vi "Chemiluminescence_VI_BM.vi"(8 "BitNum":u32, 11 "BoardNum":u32=1) -> ()   [LabVIEW 2021]
uses:
  <vilib>/ULx/Create Channel.llb/ULx Create Channel (AI-Voltage-Basic).vi
  <vilib>/ULx/Read.llb/ULx Read (Analog DBL 1Chan 1Samp).vi
  <vilib>/express/express shared/transition.llb/Dynamic To Waveform Array.vi
  <vilib>/express/express signal manip/GetorSetDDTAttributes/Set DDT Attributes/SetT0.vi
  <vilib>/express/express shared/transition.llb/Waveform Array To Dynamic.vi
  <vilib>/express/express signal manip/GetorSetDDTAttributes/Set DDT Attributes/Set DDT Properties.xnode
  <vilib>/ptbypt/NI_PtbyPt.lvlib
  <vilib>/Analysis/NI_AALBase.lvlib
panel:
  in  "Integrate Peaks":bool
  in  "Drop pt.s?":i32=1
  in  "Width":i32=6
  in  "Window (s)":dbl=5.0
  in  "Plot Type":T1(ring)=enum."Raw Data"
  in  "stop":bool
  out "Stop indicator":bool
  out "error out":errorcluster
  in  "Tab Control":enum32{"Metadata", "Detector Params", "GPS"}(tab)
  out "Time Remaining":string="11:05:15"
  out "Iteration":i32=53112
  out "JD_Second":dbl=57.335 format="%_2g"
  out "JD_Hour":dbl=13.0 format="%_2g"
  out "JD_Minute":dbl=11.0 format="%_2g"
  out "Julian Day":dbl=47.54996527777778 format="%_14g"
  out "Latitude":dbl=5158.901913
  out "Longitude":dbl=11500.024835
  out "Day":dbl=47.0 format="%#_12g"
  out "Elapsed Time (s)":dbl=17685.58402299881
  in  "Format Date":string="%d-%d-%d"
  out "Date Output":string="2024-02-16"
  in  "max V":dbl=5.0
  in  "min V":dbl=-5.0
  in  "DAQ Type":u16(ring) items=["NI DAQ", "MC DAQ"]
  in  "Sampling Frequency":dbl=3.0
  in  "device name":tag="Dev1"
  in  "Runtime Limit (mins)":dbl=960.0 format="%#_13g"
  in  "GPS\nConnected?":bool=TRUE
  in  "GPS\n 2":refnum<visa-resource-name>="COM1"
  in  "GPS Baud":dbl=4800.0
  out "GPS_Latitude":dbl=5158.901913 format="%_4g"
  out "GPS_Longitude":dbl=11500.024835 format="%_4g"
  out "GPS_jd":dbl=47.54995370370371 format="%_5g"
  out "GPS_Day":dbl=47.0
  out "GPS_Hour":dbl=13.0
  out "GPS_Minute":dbl=11.0
  out "GPS_Second":dbl=56.0
  in  "Local save location:":string="C:\\Users\\LabPC1\\OneDrive\\Desktop\\CL_Data\\MISO\\CL_test"
  in  "Cruise ID":string="MISO"
  in  "Add a comment to file (MID)":string=" "
  in  "Backup save location:":string="C:\\Users\\LabPC1\\OneDrive\\Desktop\\CL_Backup_Data\\MISO\\CL_test"
  out "Windowed SD (V)":dbl=0.038392270385846874 format="%0.2f"
  out "Windowed Mean (V)":dbl=0.04536187144435753 format="%0.2f"
  out "PMT (V)":dbl=0.0252248007909035 format="%_6g"
  out "PMT V out":cluster{"Y":dbl[], "Y":dbl[]}[](graph)
  out "Hour":dbl=13.0
  out "Minute":dbl=11.0
  out "Second":dbl=11.0
  # "DMS/O/P Chemiluminescence Program"
  # "Hz"
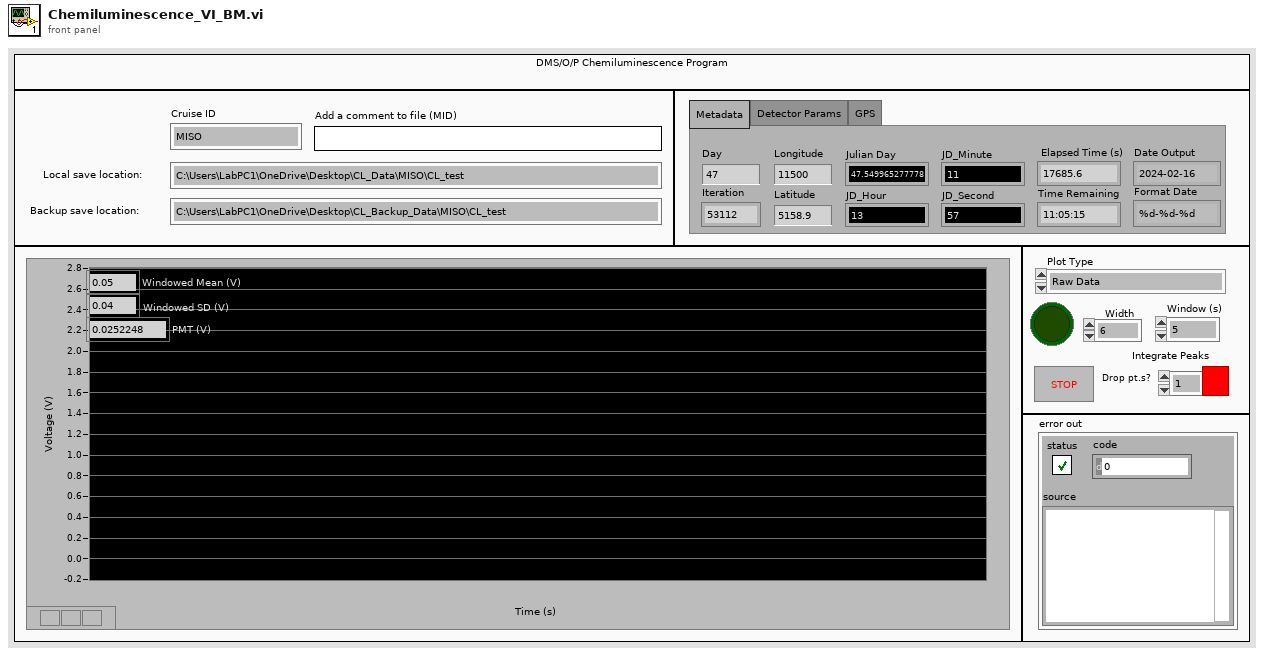
[diagram p1: front panel]
types:
  T1 = enum16{"Raw + Running Mean", "Running Mean", "Raw Data"}
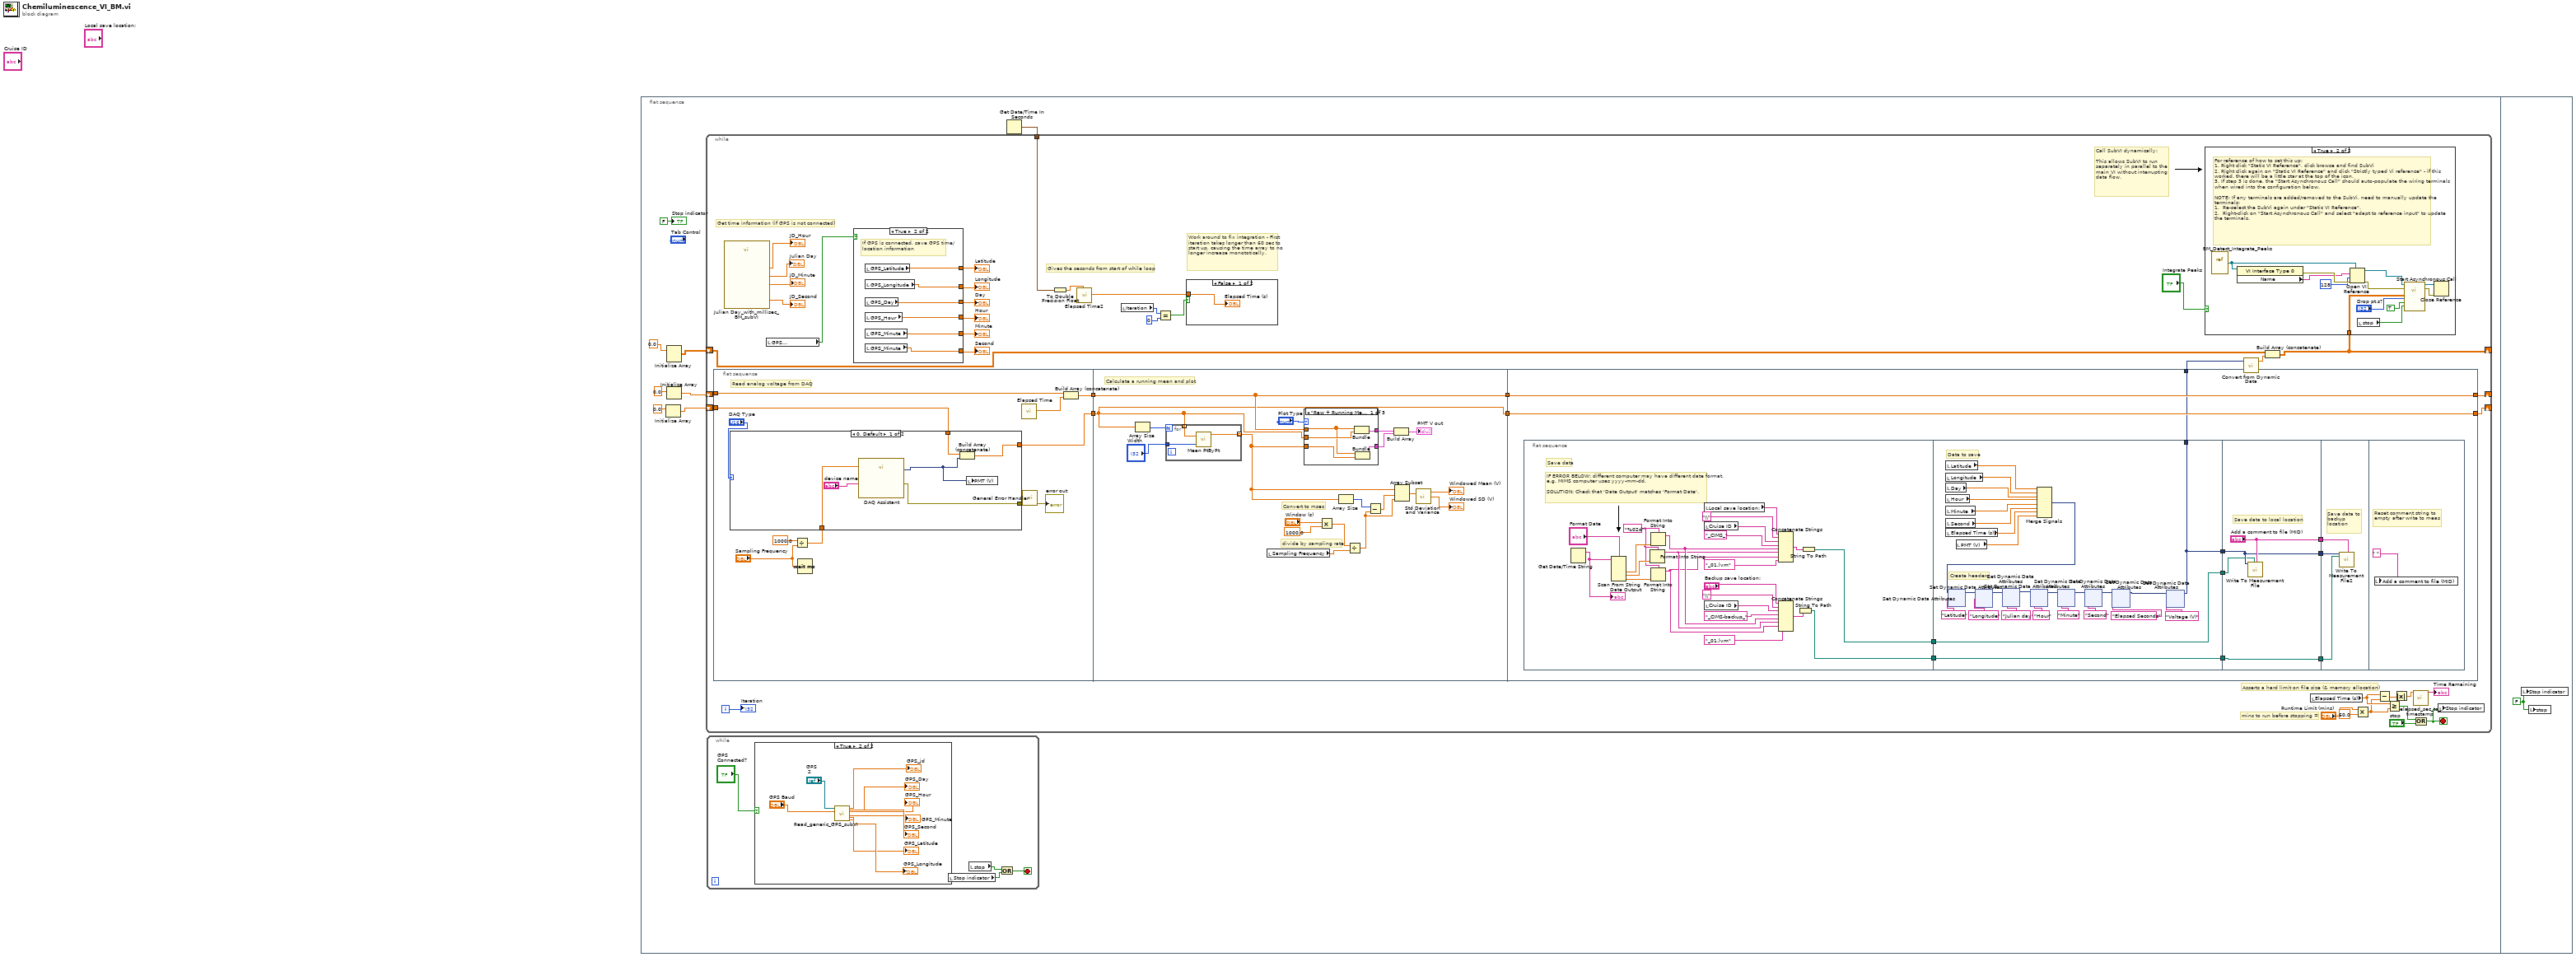
[diagram p0: block diagram]
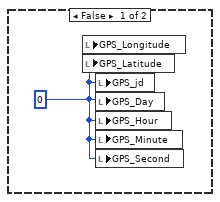
[diagram p2: hidden frame]
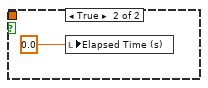
[diagram p4: hidden frame]
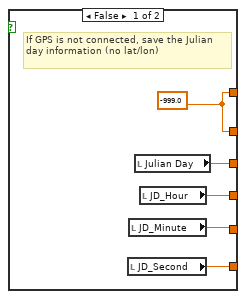
[diagram p5: hidden frame]
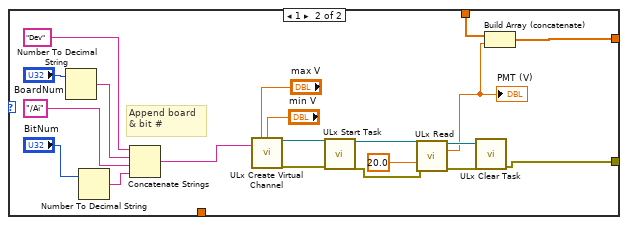
[diagram p6: hidden frame]
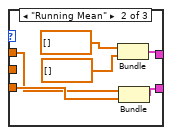
[diagram p7: hidden frame]
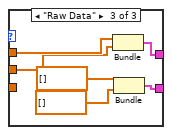
[diagram p8: hidden frame]
diagram:
  n1 = flat-sequence {
    frame #0 {
      n2 = Initialize Array(0.0 ("element")) -> (w5:dbl[])  [unwired: 1 in]
      n3 = Initialize Array(0.0 ("element")) -> (w1:dbl[][])  [unwired: 2 in]
      n4 = Initialize Array(0.0 ("element")) -> (w7:dbl[])  [unwired: 1 in]
      n5 = while {
        stop <- w10 stop-if-true
        n6 = case shown="True" "GPS\nConnected?" {
          frame False {
            w13 = 0
            n7 = local write "GPS_Longitude"(w13) -> ()
            n8 = local write "GPS_Latitude"(w13) -> ()
            n9 = local write "GPS_jd"(w13) -> ()
            n10 = local write "GPS_Day"(w13) -> ()
            n11 = local write "GPS_Hour"(w13) -> ()
            n12 = local write "GPS_Minute"(w13) -> ()
            n13 = local write "GPS_Second"(w13) -> ()
          }
          frame True {
            n14 = call "Read_generic_GPS_subVI.vi"("Baud Rate"="GPS Baud", "VISA resource name"="GPS\n 2") -> ("Longitude W"=→"GPS_Longitude":dbl, "GPS\nSeconds"=→"GPS_Second":dbl, "GPS\nHour"=→"GPS_Hour":dbl, "GPS JD"=→"GPS_jd":dbl, "Latitude N"=→"GPS_Latitude":dbl, "GPS\nDay"=→"GPS_Day":dbl, "GPS\nMinute"=→"GPS_Minute":dbl)  [unwired: 3 in]
          }
        }
        n15 = local read "Stop indicator"() -> (w9:bool)
        n16 = local read "stop"() -> (w11:bool)
        n17 = Or(x=w11, y=w9) -> (x .or. y?=w10:bool)
      }
      n18 = Get Date/Time In Seconds() -> (seconds since 1Jan1904=w4:timestamp)
      n19 = while {
        shift-right: [w28] -> _
        shift-left: w5 -> [w63]
        shift-right: [w61] -> _
        shift-left: w7 -> [w62]
        tunnel: w4 -> [w40]
        shift-right: [w23] -> _
        shift-left: w1 -> [w24]
        i -> [w32]
        stop <- w34 stop-if-true
        # "Call SubVI dynamically:\n\nThis allows SubVI to run separately in parallel to the main VI without interrupting data flow."
        # "mins to run before stopping ="
        # "Asserts a hard limit on file size (& memory allocation)"
        # "Work around to fix integration - First iteration takes longer than 60 sec to start up, causing the time array to no longer increase monototically."
        # "Gives the seconds from start of while loop"
        # "Get time information (if GPS is not connected)"
        n20 = flat-sequence {
          tunnel: w63 -> [w93]
          tunnel: w62 -> [w96]
          tunnel: [w92] -> w60
          tunnel: [w95] -> w58
          tunnel: w60 -> [w129]
          tunnel: [w129] -> w59
          tunnel: w58 -> [w143]
          tunnel: [w143] -> w57
          tunnel: [w175] -> w28
          tunnel: w59 -> [w175]
          tunnel: w57 -> [w174]
          tunnel: [w174] -> w61
          tunnel: [w165] -> w25
          frame #0 {
            # "Read analog voltage from DAQ"
            n21 = Divide(x=1000.0, y="Sampling Frequency") -> (x/y=w89:dbl)
            n22 = case shown="0, Default" "DAQ Type" {
              tunnel: [w104 w109] -> w99
              tunnel: w93 -> [w103 w108]
              tunnel: [w102 w107] -> w92
              tunnel: w89 -> [w100 _]
              frame 0, Default {
                n23 = call "DAQ Assistant"("number of samples"=w100, "device name"="device name") -> ("data"=w101:dynamicdata, "error out"=w104:errorcluster)  [unwired: 14 in, 2 out]
                n24 = Build Array (concatenate)(w103, w101) -> (w102:dbl[])
                n25 = local write "PMT (V)"(w101) -> ()
              }
              frame 1 {
                # "Append board\n& bit #"
                n26 = Number To Decimal String(number="BoardNum") -> (decimal integer string=w120:string)  [unwired: 1 in]
                n27 = Number To Decimal String(number="BitNum") -> (decimal integer string=w121:string)  [unwired: 1 in]
                n28 = Concatenate Strings("Dev", w120, "/Ai", w121) -> (w118:string)
                n29 = call-poly <vilib>:"ULx Create Virtual Channel.vi"("maximum value"="max V", "minimum value"="min V", "physical channels"=w118) -> ("task out"=w113:refnum<k24>, "error out"=w110:errorcluster)  [unwired: 11 in]
                n30 = call <vilib>:"ULx Start Task.vi"("task in"=w113, "error in"=w110) -> ("task out"=w112:refnum<k24>, "error out"=w111:errorcluster)  [unwired: 12 in]
                n31 = call-poly <vilib>:"ULx Read.vi"("task in"=w112, "timeout"=20.0, "error in"=w111) -> ("task out"=w125:refnum<k24>, "data"=w106:dbl, "error out"=w124:errorcluster)  [unwired: 10 in]
                "PMT (V)" <- w106
                n32 = call <vilib>:"ULx Clear Task.vi"("task in"=w125, "error in"=w124) -> ("error out"=w109:errorcluster)  [unwired: 13 in]
                n33 = Build Array (concatenate)(w108, w106) -> (w107:dbl[])
              }
            }
            n34 = Wait (ms)(milliseconds to wait="Sampling Frequency") -> ()  [unwired: 1 out]
            n35 = call "Elapsed Time"() -> ("Elapsed Time (s)"=w97:dbl)  [unwired: 12 in, 7 out]
            n36 = call <vilib>:"General Error Handler.vi"("error in (no error)"=w99) -> ("error out"=→"error out":errorcluster)  [unwired: 10 in, 4 out]
            n37 = Build Array (concatenate)(w96, w97) -> (w95:dbl[])
          }
          frame #1 {
            # "Calculate a running mean and plot"
            # "divide by sampling rate"
            # "Convert to msec"
            n38 = Array Size(array=w129) -> (size(s)=w131:i32)
            n39 = for {
              N: w131 -> [_]
              tunnel: [w164] -> w128 mode=indexing
              tunnel: "Width" -> [w163]
              tunnel: w129 -> [w162] mode=indexing
              n40 = call <vilib>:"Mean PtByPt.vi"("x"=w162, "sample length"=w163) -> ("mean"=w164:dbl)  [unwired: 2 in, 1 out]
            }
            n41 = local read "Sampling Frequency"() -> (w132:dbl)
            n42 = case shown="\"Raw + Running Mean\", Default" "Plot Type" {
              tunnel: w129 -> [w149 _ w158]
              tunnel: w143 -> [w148 w152 w159]
              tunnel: [w146 w150 w156] -> w127
              tunnel: w128 -> [w147 w155 _]
              tunnel: [w145 w151 w157] -> w126
              frame "Raw + Running Mean", Default {
                n43 = Bundle(w148, w149) -> (w146:cluster{dbl[], dbl[]})  [unwired: 1 in]
                n44 = Bundle(w148, w147) -> (w145:cluster{dbl[], dbl[]})  [unwired: 1 in]
              }
              frame "Running Mean" {
                n45 = Bundle(dbl[] [], dbl[] []) -> (w150:cluster{dbl[], dbl[]})  [unwired: 1 in]
                n46 = Bundle(w152, w155) -> (w151:cluster{dbl[], dbl[]})  [unwired: 1 in]
              }
              frame "Raw Data" {
                n47 = Bundle(w159, w158) -> (w156:cluster{dbl[], dbl[]})  [unwired: 1 in]
                n48 = Bundle(dbl[] [], dbl[] []) -> (w157:cluster{dbl[], dbl[]})  [unwired: 1 in]
              }
            }
            n49 = Multiply(x="Window (s)", y=1000.0) -> (x*y=w139:dbl)
            n50 = Array Size(array=w128) -> (size(s)=w141:i32)
            n51 = Divide(x=w139, y=w132) -> (x/y=w137:dbl)
            n52 = Subtract(x=w141, y=w137) -> (x-y=w133:dbl)
            n53 = Build Array(w127, w126) -> (→"PMT V out":cluster{dbl[], dbl[]}[])
            n54 = Array Subset(array=w128, index=w133, length=w137) -> (w130:dbl[])
            n55 = call <vilib>:"Std Deviation and Variance.vi"("X"=w130) -> ("mean"=→"Windowed Mean (V)":dbl, "standard deviation"=→"Windowed SD (V)":dbl)  [unwired: 1 in, 1 out]
          }
          frame #2 {
            n56 = flat-sequence {
              tunnel: [w177] -> w173
              tunnel: [w176] -> w172
              tunnel: [w199] -> w171
              tunnel: w173 -> [w213]
              tunnel: [w213] -> w170
              tunnel: [w200] -> w169
              tunnel: w172 -> [w200]
              tunnel: [w199] -> w165
              tunnel: ["Add a comment to file (MID)"] -> w168
              tunnel: w171 -> [w340]
              tunnel: [w340] -> w167
              tunnel: w170 -> [w339]
              tunnel: w169 -> [w338]
              tunnel: [w338] -> w166
              tunnel: w168 -> [w344]
              tunnel: w167 -> [w343]
              tunnel: w166 -> [w342]
              frame #0 {
                w178 = "%02d"
                # "IF ERROR BELOW: different computer may have different date format, e.g. MIMS computer uses yyyy-mm-dd.\n\nSOLUTION: Check that 'Date Output' matches 'Format Date'."
                # "Save data"
                n57 = Get Date/Time String() -> (date string=w198:string)  [unwired: 3 in, 1 out]
                "Date Output" <- w198
                n58 = Scan From String(format string="Format Date", input string=w198) -> (output 1=w197:dbl, output 2=w196:dbl, output 3=w195:dbl)  [unwired: 5 in, 3 out]
                n59 = Format Into String(format string=w178, w196) -> (resulting string=w187:string)  [unwired: 2 in, 1 out]
                n60 = Format Into String(format string=w178, w197) -> (resulting string=w188:string)  [unwired: 2 in, 1 out]
                n61 = Format Into String(format string=w178, w195) -> (resulting string=w186:string)  [unwired: 2 in, 1 out]
                n62 = local read "Local save location:"() -> (w194:string)
                n63 = local read "Cruise ID"() -> (w193:string)
                n64 = local read "Cruise ID"() -> (w192:string)
                n65 = Concatenate Strings(w194, "\\", w193, "_CIMS_", w188, w187, w186, "_01.lvm") -> (w191:string)
                n66 = Concatenate Strings("Backup save location:", "\\", w192, "_CIMS-backup_", w188, w187, w186, "_01.lvm") -> (w190:string)
                n67 = String To Path(string=w190) -> (path=w176:path)
                n68 = String To Path(string=w191) -> (path=w177:path)
              }
              frame #1 {
                # "Data to save"
                # "Create headers"
                n69 = local read "Latitude"() -> (w209:dbl)
                n70 = local read "Longitude"() -> (w208:dbl)
                n71 = local read "Day"() -> (w207:dbl)
                n72 = local read "Hour"() -> (w206:dbl)
                n73 = local read "Minute"() -> (w205:dbl)
                n74 = local read "Second"() -> (w204:dbl)
                n75 = local read "Elapsed Time (s)"() -> (w202:dbl)
                n76 = local read "PMT (V)"() -> (w203:dbl)
                n77 = Merge Signals(w209, w208, w207, w206, w205, w204, w202, w203) -> (w201:dynamicdata)
                n78 = xnode ("Set Dynamic Data Attributes")("Signals In"=w201, "Signal Name"="Latitude") -> ("Signals Out"=w218:dynamicdata)  [unwired: 2 in, 1 out]
                n79 = xnode ("Set Dynamic Data Attributes")("Signals In"=w218, "Signal Name"="Longitude") -> ("Signals Out"=w217:dynamicdata)  [unwired: 2 in, 1 out]
                n80 = xnode ("Set Dynamic Data Attributes")("Signals In"=w217, "Signal Name"="Julian day") -> ("Signals Out"=w216:dynamicdata)  [unwired: 2 in, 1 out]
                n81 = xnode ("Set Dynamic Data Attributes")("Signals In"=w216, "Signal Name"="Hour") -> ("Signals Out"=w215:dynamicdata)  [unwired: 2 in, 1 out]
                n82 = xnode ("Set Dynamic Data Attributes")("Signals In"=w215, "Signal Name"="Minute") -> ("Signals Out"=w214:dynamicdata)  [unwired: 2 in, 1 out]
                n83 = xnode ("Set Dynamic Data Attributes")("Signals In"=w214, "Signal Name"="Second") -> ("Signals Out"=w212:dynamicdata)  [unwired: 2 in, 1 out]
                n84 = xnode ("Set Dynamic Data Attributes")("Signals In"=w212, "Signal Name"="Elapsed Seconds") -> ("Signals Out"=w211:dynamicdata)  [unwired: 2 in, 1 out]
                n85 = xnode ("Set Dynamic Data Attributes")("Signals In"=w211, "Signal Name"="Voltage (V)") -> ("Signals Out"=w199:dynamicdata)  [unwired: 2 in, 1 out]
              }
              frame #2 {
                # "Save data to local location"
                n86 = call "Write To Measurement File"("Signals"=w340, "Filename"=w339, "Comment"="Add a comment to file (MID)") -> ()  [unwired: 14 in, 3 out]
              }
              frame #3 {
                # "Save data to backup location"
                n87 = call "Write To Measurement File2"("Signals"=w343, "Filename"=w342, "Comment"=w344) -> ()  [unwired: 14 in, 3 out]
              }
              frame #4 {
                # "Reset comment string to empty after write to meas"
                n88 = local write "Add a comment to file (MID)"(" " ("Add a comment to file (MID)")) -> ()
              }
            }
          }
        }
        n89 = call "Julian Day_with_millisec_BM_subVI.vi"() -> ("Julian Day"=→"Julian Day":dbl, "hour"=→"JD_Hour":dbl, "minute"=→"JD_Minute":dbl, "Decimal second"=→"JD_Second":dbl)  [unwired: 11 in, 1 out]
        n90 = local read "GPS\nConnected?"() -> (w50:bool)
        n91 = case shown="True" w50 {
          tunnel: [w78 w88] -> w56
          tunnel: [w79 w87] -> w55
          tunnel: [w80 w86] -> w54
          tunnel: [w81 w85] -> w53
          tunnel: [w82 w84] -> w52
          tunnel: [w82 w83] -> w51
          frame False {
            w82 = -999.0 ("GPS_Latitude")
            # "If GPS is not connected, save the Julian day information (no lat/lon)"
            n92 = local read "JD_Second"() -> (w78:dbl)
            n93 = local read "JD_Minute"() -> (w79:dbl)
            n94 = local read "Julian Day"() -> (w81:dbl)
            n95 = local read "JD_Hour"() -> (w80:dbl)
          }
          frame True {
            # "If GPS is connected, save GPS time/location information"
            n96 = local read "GPS_Latitude"() -> (w83:dbl)
            n97 = local read "GPS_Longitude"() -> (w84:dbl)
            n98 = local read "GPS_Day"() -> (w85:dbl)
            n99 = local read "GPS_Hour"() -> (w86:dbl)
            n100 = local read "GPS_Minute"() -> (w87:dbl)
            n101 = local read "GPS_Minute"() -> (w88:dbl)
          }
        }
        "Latitude" <- w51
        "Longitude" <- w52
        "Day" <- w53
        "Hour" <- w54
        "Minute" <- w55
        "Second" <- w56
        n102 = To Double Precision Float(number=w40) -> (double precision float=w45:dbl)
        n103 = call "Elapsed Time2"("Set Start Time (s)"=w45) -> ("Elapsed Time (s)"=w42:dbl)  [unwired: 11 in, 7 out]
        n104 = local read "Iteration"() -> (w43:i32)
        n105 = Equal?(x=w43, y=0) -> (x = y?=w44:bool)
        n106 = case shown="False" w44 {
          tunnel: w42 -> [w76 _]
          frame False {
            "Elapsed Time (s)" <- w76
          }
          frame True {
            n107 = local write "Elapsed Time (s)"(0.0 ("Elapsed Time (s)")) -> ()
          }
        }
        n108 = call "Convert from Dynamic Data"("Dynamic Data Type"=w25) -> ("Array"=w26:dbl[])  [unwired: 3 in]
        n109 = Build Array (concatenate)(w24, w26) -> (w23:dbl[][])
        n110 = case shown="True" "Integrate Peaks" {
          tunnel: w23 -> [_ w68]
          frame False {
          }
          frame True {
            # "For reference of how to set this up:\n1. Right click \"Static VI Reference\", click browse and find SubVi\n2. Right click again on \"Static VI Reference\" and click \"Strictly typed Vi reference\" - if this worked, there will be a little star at the top of the icon.\n3. If step 3 is done, the \"Start Asynchronous Call\" should auto-populate the wiring terminals when wired into the configuration below.\n\nNOTE: If any terminals are added/removed to the SubVi, need to manually update the terminals:\n1.  Re-select the SubVi again under \"Static VI Reference\".\n2.  Right-click on \"Start Asynchronous Call\" and select \"adapt to reference input\" to update the terminals."
            n111 = vi-ref "BM_Detect_Integrate_Peaks.vi"() -> (w71:refnum<vi>)
            n112 = property class="VI Interface Type 0"(reference=w71) -> (error out=w75:errorcluster, "Name"=w74:string)  [unwired: 1 in, 1 out]
            n113 = Open VI Reference(type specifier VI Refnum (for type only)=w71, vi path=w74, options=128, error in (no error)=w75) -> (vi reference=w69:refnum<vi>, error out=w70:errorcluster)  [unwired: 2 in]
            n114 = local read "stop"() -> (w72:bool)
            n115 = call-by-ref "Start Asynchronous Call"(reference=w69, error in=w70, "stop"=w72, "Use as SubVI?"=TRUE, "Drop pt.s?"="Drop pt.s?", "Imported Data"=w68) -> (reference out=w64:refnum<vi>, error out=w65:errorcluster)  [unwired: 6 in, 2 out]
            n116 = Close Reference(reference=w64, error in (no error)=w65) -> ()  [unwired: 1 out]
          }
        }
        n117 = local read "Elapsed Time (s)"() -> (w38:dbl)
        n118 = Multiply(x="Runtime Limit (mins)", y=60.0) -> (x*y=w37:dbl)
        n119 = Subtract(x=w38, y=w37) -> (x-y=w31:dbl)
        n120 = Greater Or Equal?(x=w38, y=w37) -> (x >= y?=w39:bool)
        n121 = Absolute Value(x=w31) -> (abs(x)=w30:dbl)
        n122 = call "elapsed_sec_to_timestamp.vi"("Input Elapsed Seconds"=w30) -> ("Timestamp"=→"Time Remaining":string)  [unwired: 10 in]
        n123 = Compound Arithmetic op=OR(w39, "stop") -> (w34:bool)
        n124 = local write "Stop indicator"(w34) -> ()
        "Iteration" <- w32
      }
      "Stop indicator" <- FALSE ("Other stop")
    }
    frame #1 {
      w346 = FALSE ("stop")
      n125 = local write "Stop indicator"(w346) -> ()
      n126 = local write "stop"(w346) -> ()
    }
  }
